vi "Query DMRS For Mapping Type A.vi"(7 "Bandwidth Part (BWP0)":T2 items=["BWP0"], 8 "error in (no error)":errorcluster, 9 "Carrier Component (1)":T1=1, 10 "Instance (1)":T3=1, 11 "VISA resource name":refnum<visa-resource-name>) -> (0 "error out":errorcluster, 1 "Config Type":i32=1, 2 "Additional Position":i32=2, 3 "VISA resource name out":refnum<visa-resource-name>, 4 "Max Length":i32=1)   [LabVIEW 2015, in "Rohde&Schwarz CMXP NR FR2 Measurement.lvlib"]
doc: "Queries the DM-RS for mapping type A.\n\nAttribute:\n-\n\nRemote-control command:\nCONFigure:NRMMw:MEAS<i>[:CC<no>]:BWPart:PUSCh:DMTA? <BWP>"
uses:
  <instrlib>/Rohde&Schwarz CMXP NR FR2 Measurement/Rohde&Schwarz CMXP NR FR2 Measurement.lvlib
  <instrlib>/Rohde&Schwarz CMXP NR FR2 Measurement/Private/_Instance.ctl
  <instrlib>/Rohde&Schwarz CMXP NR FR2 Measurement/Private/_Bandwidth Part.ctl
  <instrlib>/Rohde&Schwarz CMXP NR FR2 Measurement/Private/_Carrier Component.ctl
  <instrlib>/Rohde&Schwarz CMXP NR FR2 Measurement/Private/rsidr_core.llb/rsidr_core.lvlib
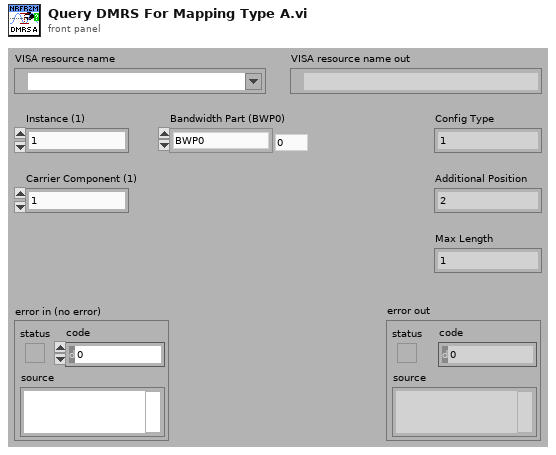
[diagram p1: front panel]
types:
  T1 = typedef "Rohde&Schwarz CMXP NR FR2 Measurement.lvlib/_Carrier Component.ctl" = i32
  T2 = typedef "Rohde&Schwarz CMXP NR FR2 Measurement.lvlib/_Bandwidth Part.ctl" = i32
  T3 = typedef "Rohde&Schwarz CMXP NR FR2 Measurement.lvlib/_Instance.ctl" = i32
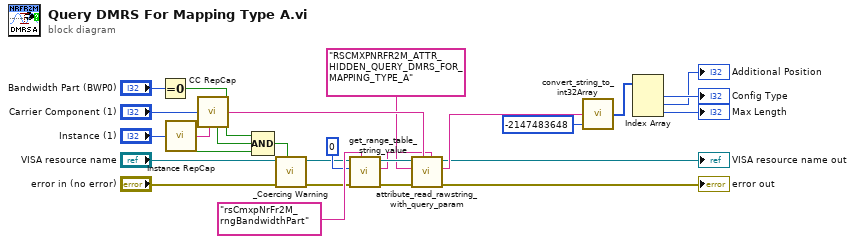
[diagram p0: block diagram]
diagram:
  n1 = Equal To 0?(x="Bandwidth Part (BWP0)") -> (x = 0?=w4:bool)
  n2 = call <instrlib>:"Instance RepCap.vi"("Instance In"="Instance (1)") -> ("In Range?"=w21:bool, "RepCap Identifier Out"=w2:string)  [unwired: 1 in]
  n3 = call <instrlib>:"CC RepCap.vi"("CC In"="Carrier Component (1)", "RepCap String In (\"\")"=w2) -> ("In Range?"=w20:bool, "RepCap Identifier Out"=w14:string)
  n4 = Compound Arithmetic op=AND(w4, w20, w21) -> (w23:bool)
  n5 = call <instrlib>:"_Coercing Warning.vi"("In Range?"=w23, "error in (no error)"="error in (no error)", "VISA resource name"="VISA resource name") -> ("error out"=w17:errorcluster, "VISA resource name out"=w18:refnum<visa-resource-name>)  [unwired: 7 in]
  n6 = call <instrlib>:"get_range_table_string_value.vi"("Range Table ID in"="rsCmxpNrFr2M_rngBandwidthPart", "error in"=w17, "I32 input"=0, "VISA resource name"=w18) -> ("error out"=w16:errorcluster, "String Value out"=w12:string, "VISA resource name out"=w15:refnum<visa-resource-name>)  [unwired: 5 in]
  n7 = call <instrlib>:"attribute_read_rawstring_with_query_param.vi"("Query Parameter (None)"=w12, "Repeated Capability"=w14, "error in"=w16, "Attribute ID"="RSCMXPNRFR2M_ATTR_HIDDEN_QUERY_DMRS_FOR_MAPPING_TYPE_A", "VISA resource name"=w15) -> ("error out"=→"error out":errorcluster, "Raw String out"=w11:string, "VISA resource name out"=→"VISA resource name out":refnum<visa-resource-name>)  [unwired: 4 in]
  n8 = call <instrlib>:"convert_string_to_int32Array.vi"("default (0)"=-2147483648, "string in"=w11) -> ("int32 array out"=w10:i32[])  [unwired: 2 in, 1 out]
  n9 = Index Array(array=w10) -> (element #1=→"Config Type":i32, element #2=→"Additional Position":i32, element #3=→"Max Length":i32)  [unwired: 3 in]
